vi "TEST_L0_MAJnADDS_(4TH)_NEW.vi"(5 "threshold":i32[][](array[numeric])=[[518, 513, 533, 498, 543, 508, 548], [526, 521, 546, 506, 551, 516, 556], [534, 529, 549, 514, 559, 524, 564], [542, 537, 557, 522, 567, 532, 572], [545, 540, 565, 530, 575, 530, 575]], 7 "Serial Number":string="testFile", 8 "error in (no error)":errorcluster, 11 "Instrument VISA in":T1={"AWG VISA"="AgilentGen1", "Oscilloscope  VISA "="AgilentOsc", "Integration Board IP"="172.16.17.47", "connection ID"=refnum, "report out"=refnum, "report file path"=path "C:/Users/omartinez/Desktop/L0nL1_Results"}) -> (0 "error out":errorcluster, 3 "Instrument VISA out":T1={"AWG VISA"="AgilentGen1", "Oscilloscope  VISA "="AgilentOsc", "Integration Board IP"="172.16.7.47", "connection ID"=refnum, "report out"=refnum, "report file path"=path "C:/Users/omartinez/Desktop/L0nL1_Results"})   [LabVIEW 2012]
uses:
  <vilib>/Utility/NIReport.llb/NI_report.lvclass
  <vilib>/Utility/NIReport.llb/HTML/NI_HTML.lvclass
  <instrlib>/Agilent 8000 Series/Public/Configure/Configure Math (Binary Operation).vi
  L0&L1/L0_BOARD_TESTs/trunk/Sum_Abrilader/L0_Sum_Adder Folder/C/Program Files/National Instruments/LabVIEW 2012/instr.lib/Agilent 8000 Series/Public/Data/Low Level/Fetch Measurement (More).vi
  <instrlib>/Agilent 8000 Series/Agilent 8000 Series.lvlib
panel:
  in  "Voltages comprobation":dbl[](array[numeric])=[0.05, 0.2]
  in  "Channels \nCombinations":i32[](array[numeric])=[3, 12, 48, 96, 7, 28, 112, 15, 120, 31, 124, 63, 126, 127]
  in  "Voltages":dbl[](array[numeric])=[0.05, 0.2]
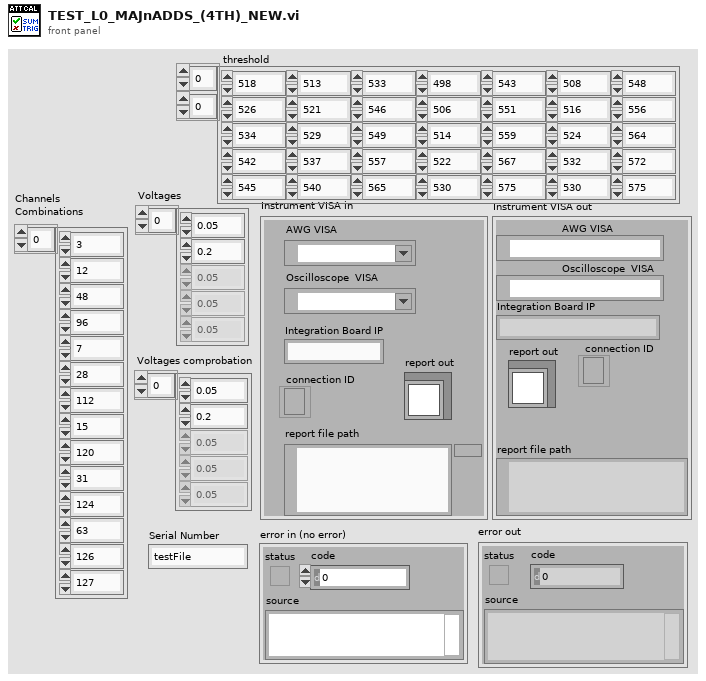
[diagram p1: front panel]
types:
  T1 = cluster{"AWG VISA":refnum<visa-resource-name>, "Oscilloscope  VISA ":refnum<visa-resource-name>, "Integration Board IP":string, "connection ID":refnum<k5>, "report out":refnum<class "NI_report.lvclass">, "report file path":path}
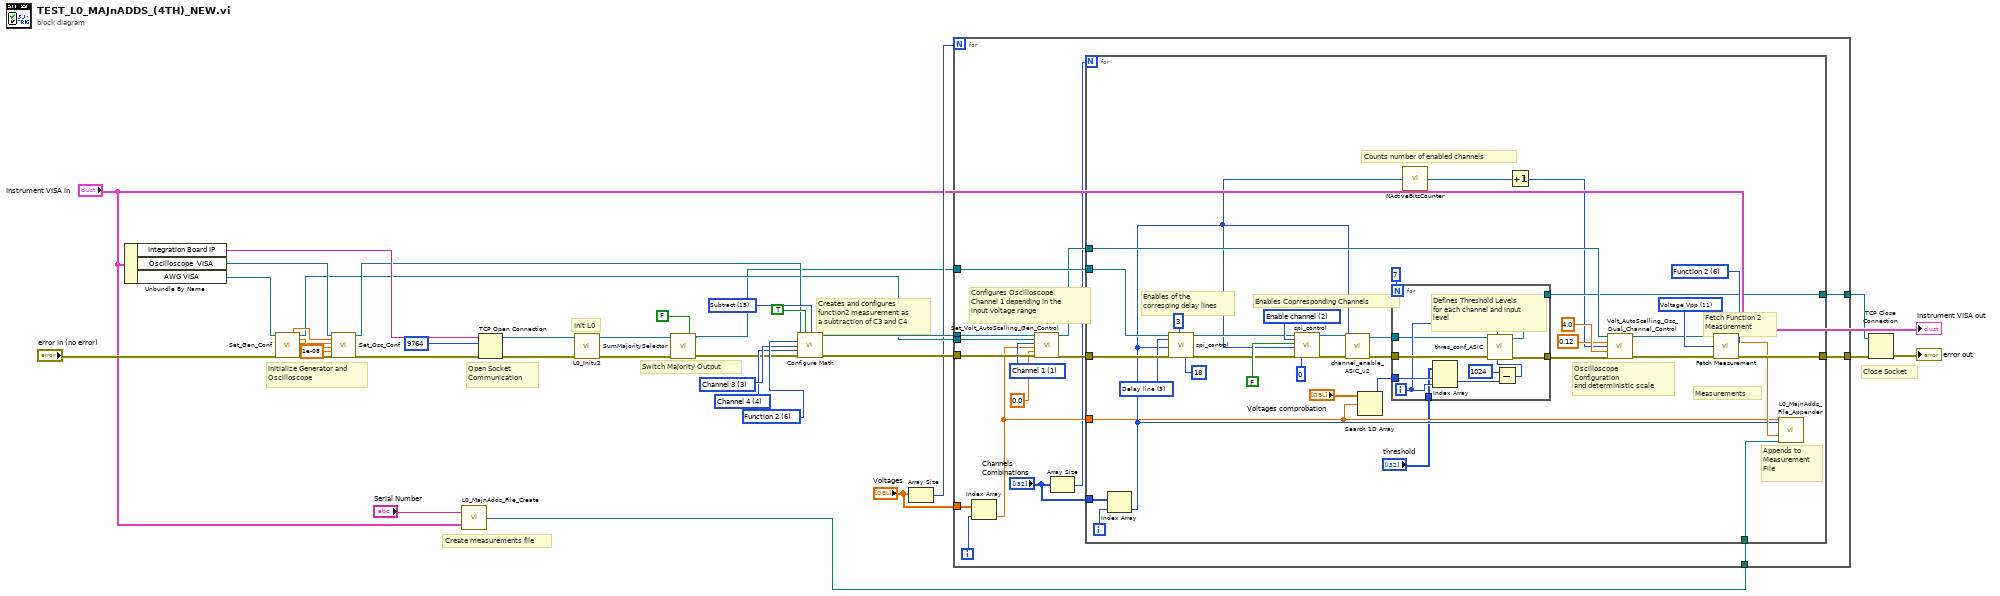
[diagram p0: block diagram]
diagram:
  w32 = u16 6 items=["Function 1"=5, "Function 2"=6, "Function 3"=7, "Function 4"=8] ("Math Channel (5: Function 1)")
  w33 = u16 15 items=["Add"=12, "Divide"=13, "Multiply"=14, "Subtract"=15, "Common Mode"=16, "Versus"=17] ("Math Operation (12: Add)")
  w31 = 3 items=["Channel 1"=1, "Channel 2"=2, "Channel 3"=3, "Channel 4"=4] ("Channel (1: Channel 1)")
  w30 = 4 items=["Channel 1"=1, "Channel 2"=2, "Channel 3"=3, "Channel 4"=4] ("Channel (1: Channel 1)")
  # "Close Socket"
  # "Create measurements file"
  # "Init L0"
  # "Switch Majority Output"
  # "Initialize Generator and \nOscilloscope"
  # "Creates and configures\nfunction2 measurement as\na subtraction of C3 and C4"
  # "Open Socket\nCommunication"
  n1 = Unbundle By Name("Instrument VISA in") -> ("Integration Board IP"=w28:string, "Oscilloscope  VISA"=w19:refnum<visa-resource-name>, "AWG VISA"=w20:refnum<visa-resource-name>)
  n2 = call "Set_Gen_Conf.vi"("AWG VISA"=w20, "error in (no error)"="error in (no error)") -> ("Amplitude 1 OUT"=w25:dbl, "VISA resource name out"=w17:refnum<visa-resource-name>, "Pulse Width in seconds 1 OUT"=w24:dbl, "Trigger Level 1"=w23:dbl, "error out"=w26:errorcluster)  [unwired: 10 in, 3 out]
  n3 = call "Set_Osc_Conf.vi"("VISA resource name"=w19, "Amplitude IN"=w25, "Trigger Level IN"=w23, "Pulse Width in seconds IN"=w24, "Position 1"=1e-08, "error in (no error)"=w26) -> ("VISA resource name out"=w18:refnum<visa-resource-name>, "error out"=w21:errorcluster)  [unwired: 12 in]
  n4 = call "L0_MajnAdds_File_Create.vi"("input cluster"="Instrument VISA in", "Serial Number"="Serial Number") -> ("appended path"=w11:path)
  n5 = TCP Open Connection(address=w28, remote port or service name=u16 9764, error in (no error)=w21) -> (connection ID=w4:refnum<k5>, error out=w7:errorcluster)  [unwired: 2 in]
  n6 = call "L0_Initv2.vi"("error in"=w7, "connection ID in"=w4) -> ("error out"=w10:errorcluster, "connection ID out"=w9:refnum<k5>)  [unwired: 8 in]
  n7 = call "SumMajoritySelector.vi"("On Sum\nOff Majority"=FALSE ("On Sum\nOff Majority"), "error in (no error)"=w10, "connection ID"=w9) -> ("error out"=w6:errorcluster, "connection ID out"=w5:refnum<k5>)  [unwired: 5 in]
  n8 = call-poly <instrlib>:"Configure Math.vi"("VISA resource name"=w18, "Enable Math Channel (T:Enable)"=TRUE, "Math Operation (12: Add)"=w33, "Math Channel (5: Function 1)"=w32, "Math Operand (1: Channel 1)"=w31, "Math Operand (2: Channel 2)"=w30, "error in (no error)"=w6) -> ("VISA resource name out"=w27:refnum<visa-resource-name>, "error out"=w29:errorcluster)  [unwired: 7 in]
  n9 = Array Size(array="Voltages") -> (size(s)=w15:i32)
  n10 = for {
    N: w15 -> [_]
    tunnel: w29 -> [w51]
    tunnel: w5 -> [w50]
    tunnel: [w49] -> w3
    tunnel: w27 -> [w48]
    tunnel: w17 -> [w47]
    tunnel: "Voltages" -> [w42]
    tunnel: w11 -> [w37]
    tunnel: [w36] -> w1
    i -> [w41]
    w46 = 1 items=["Channel 1"=1, "Channel 2"=2, "Channel 3"=3, "Channel 4"=4] ("Channel")
    # "Configures Oscilloscope\nChannel 1 depending in the \ninput voltage range"
    n11 = Index Array(array=w42, index=w41) -> (element=w40:dbl)
    n12 = call "Set_Volt_AutoScalling_Gen_Control.vi"("VISA Oscilloscope"=w48, "VISA Generator"=w47, "Channel"=w46, "Amplitude"=w40, "DC Offset"=0.0, "error in (no error)"=w51) -> ("VISA Oscilloscope"=w43:refnum<visa-resource-name>, "error out"=w44:errorcluster)  [unwired: 11 in, 1 out]
    n13 = Array Size(array="Channels \nCombinations") -> (size(s)=w38:i32)
    n14 = for {
      N: w38 -> [_]
      tunnel: w50 -> [w87]
      tunnel: [w68] -> w49
      tunnel: w44 -> [w86]
      tunnel: w43 -> [w85]
      tunnel: w40 -> [w62]
      tunnel: "Channels \nCombinations" -> [w73]
      tunnel: w37 -> [w65]
      tunnel: [w56] -> w36
      i -> [w72]
      w71 = 11 items=["Rise Time", "Fall Time", "Frequency", "Period", "Voltage RMS(AC)", "Voltage RMS(DC)", "Voltage RMS (AC,cycle)", "Voltage RMS (DC,cycle)", "Voltage Max", "Voltage Min", "Voltage Middle", "Voltage Vpp", "Voltage High", "Voltage Low", "Voltage Average", "Voltage Average (cycle)", "Width Negative", "Width Positive", "Duty Cycle Positive", "Amplitude", "Overshoot", "Preshoot", "Voltage Base", "Voltage Upper", "Time Max", "Time Min", "Color Grade Crossing", "Color Grade Eye Width", "Color Grade Eye Height", "Color Grade Eye Q-Factory", "Color Grade Eye Duty Cycle Distortion(Percent)", "Color Grade Eye Duty Cycle Distortion(Time)", "Color Grade Eye Jitter(PP)", "Color Grade Eye Width(RMS)", "Cycle-cycle Duty Jitter(Rising)", "Cycle-cycle Duty Jitter(Falling)", "Cycle-cycle Jitter(Rising)", "Cycle-cycle Jitter(Falling)", "Cycle-cycle - Width", "Cycle-cycle + Width", "Date Rate", "Unit Interval", "FFT Delta Frequency", "FFT Delta Magnitude", "FFT Frequency", "FFT Magnitude", "Slew Rate", "Area (Entire Display)", "Area(Single Cycle)", "Duty Cycle (Rising)", "Duty Cycle (Falling)"] ("Measurement Function (0: Rise Time)")
      w70 = 6 items=["Channel 1"=1, "Channel 2"=2, "Channel 3"=3, "Channel 4"=4, "Function 1"=5, "Function 2"=6, "Function 3"=7, "Function 4"=8, "Memory 1"=9, "Memory 2"=10, "Memory 3"=11, "Memory 4"=12] ("Channel (1: Channel 1)")
      w79 = u16 2 items=["Attenuation", "Clipping", "Enable channel", "Delay line", "ASIC"] ("Device")
      w81 = u16 3 items=["Attenuation", "Clipping", "Enable channel", "Delay line", "ASIC"] ("Device")
      # "Appends to\nMeasurement\nFile"
      # "Counts number of enabled channels"
      # "Fetch Function 2\nMeasurement"
      # "Measurements"
      # "Enables of the\ncorresping delay lines"
      # "Enables Coprresponding Channels"
      # "Oscilloscope Configuration \nand deterministic scale"
      n15 = Index Array(array=w73, index=w72) -> (element=w64:i32)
      n16 = call "spi_control.vi"("connection ID"=w87, "Device"=w81, "Data"=w64, "Register or channel"=18, "error in"=w86, "chip delay"=3) -> ("connection ID out"=w77:refnum<k5>, "error out 2"=w76:errorcluster)  [unwired: 6 in, 6 out]
      n17 = call "spi_control.vi"("connection ID"=w77, "Device"=w79, "Read/#write"=FALSE, "Data"=w64, "error in"=w76, "Id in"=0) -> ("connection ID out"=w75:refnum<k5>, "error out 2"=w74:errorcluster)  [unwired: 6 in, 6 out]
      n18 = call "channel_enable_ASIC_v2.vi"("error in"=w74, "Channel Combination"=w64, "Connection ID in"=w75) -> ("error out"=w59:errorcluster, "Connection ID out"=w58:refnum<k5>)  [unwired: 7 in]
      n19 = Search 1D Array(1D array="Voltages comprobation", element=w62) -> (index of element=w61:i32)  [unwired: 1 in]
      n20 = for {
        N: 7 -> [_]
        tunnel: w61 -> [w96]
        tunnel: w59 -> [w97]
        tunnel: w58 -> [w94]
        tunnel: [w93] -> w57
        tunnel: [w92] -> w56
        tunnel: "threshold" -> [w91]
        i -> [w95]
        # "Defines Threshold Levels\nfor each channel and input\nlevel"
        n21 = Index Array(array=w91, index (row)=w96, index (col)=w95) -> (element=w90:i32)
        n22 = Subtract(x=1024, y=w90) -> (x-y=w89:i32)
        n23 = call "thres_conf_ASIC.vi"("threshold"=w89, "Ring"=w95, "error out 3"=w97, "connection ID"=w94) -> ("error out 2"=w93:errorcluster, "connection ID out"=w92:refnum<k5>)  [unwired: 4 in, 2 out]
      }
      n24 = call "NActiveBitsCounter.vi"("Input Number"=w64) -> ("N High Bits"=w53:i32)
      n25 = Increment(x=w53) -> (x+1=w52:i32)
      n26 = call "Volt_AutoScalling_Osc_Dual_Channel_Control.vi"("VISA Oscilloscope"=w85, "Voltage In"=0.12, "N Channels"=w52, "Offset Divider"=4.0, "error in"=w57) -> ("VISA resource name out"=w67:refnum<visa-resource-name>, "error out"=w69:errorcluster)  [unwired: 9 in]
      n27 = call-poly "Fetch Measurement.vi"("VISA resource name"=w67, "Channel (1: Channel 1)"=w70, "Measurement Function (0: Rise Time)"=w71, "error in (no error)"=w69) -> ("Measurement"=w66:dbl, "error out"=w68:errorcluster)  [unwired: 9 in, 1 out]
      n28 = call "L0_MajnAdds_File_Appender.vi"("Vin"=w62, "CH"=w64, "Vmeas"=w66, "file path (dialog if empty)"=w65) -> ()  [unwired: 24 in]
    }
  }
  n29 = TCP Close Connection(connection ID=w1, error in (no error)=w3) -> (error out=→"error out":errorcluster)  [unwired: 1 in, 1 out]
  "Instrument VISA out" <- "Instrument VISA in"
